vi "Kaelus SWI Set Stimulus.vi"(7 "Kaelus SWI":T4, 8 "error in (no error)":errorcluster, 10 "SWI Position":T1, 11 "DAQmx Dev Name (SWModule)":string) -> (0 "error out":errorcluster, 3 "DAQmx Dev Name (SWModule)":string)   [LabVIEW 2011]
uses:
  TypeDefs/Kaelus SWI Instrument Info.ctl
  TypeDefs/Kaelus SWI Position.ctl
  BPIMCore EXT/WebEngine/LIB/MODULES/SW Module/SW Tx Positions.ctl
  BPIMCore EXT/WebEngine/LIB/MODULES/SW Module/SW Rx Positions.ctl
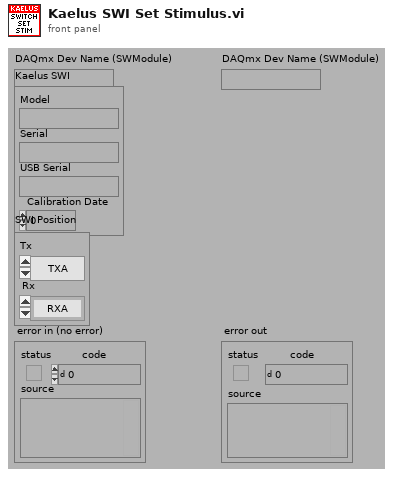
[diagram p1: front panel]
types:
  T1 = typedef "Kaelus SWI Position.ctl" = cluster{"Tx":T2, "Rx":T3}
  T2 = typedef "SW Tx Positions.ctl" = enum16{"TXA", "TXB", "TXC"}
  T3 = typedef "SW Rx Positions.ctl" = enum16{"RXA", "RXB", "RXC", "RXD", "RXE", "RXF"}
  T4 = typedef "Kaelus SWI Instrument Info.ctl" = cluster{"Model":string, "Serial":string, "USB Serial":string, "Calibration Date":dbl}
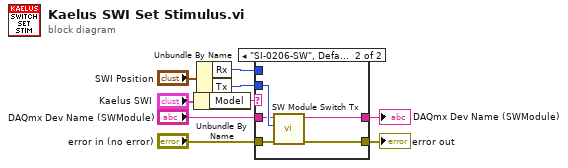
[diagram p0: block diagram]
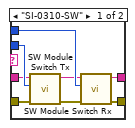
[diagram p2: hidden frame]
diagram:
  n1 = Unbundle By Name("Kaelus SWI") -> ("Model"=w5:string)
  n2 = Unbundle By Name("SWI Position") -> ("Rx"=w3:T3, "Tx"=w2:T2)
  n3 = case shown="\"SI-0206-SW\", Default" w5 {
    tunnel: "error in (no error)" -> [w14 w19]
    tunnel: [w13 w17] -> w8
    tunnel: "DAQmx Dev Name (SWModule)" -> [w10 w16]
    tunnel: w3 -> [w12 _]
    tunnel: w2 -> [w11 w18]
    tunnel: [w10 w16] -> w1
    frame "SI-0310-SW" {
      n4 = call "SW Module Switch Tx.vi"("error in (no error)"=w14, "Tx Position"=w11, "SW Dmx Name"=w10) -> ("error out"=w15:errorcluster)  [unwired: 8 out]
      n5 = call "SW Module Switch Rx.vi"("error in (no error)"=w15, "Rx Position"=w12, "SW Dmx Name"=w10) -> ("error out"=w13:errorcluster)  [unwired: 8 out]
    }
    frame "SI-0206-SW", Default {
      n6 = call "SW Module Switch Tx.vi"("error in (no error)"=w19, "Tx Position"=w18, "SW Dmx Name"=w16) -> ("error out"=w17:errorcluster)  [unwired: 8 out]
    }
  }
  "error out" <- w8
  "DAQmx Dev Name (SWModule)" <- w1
